vi "SCADA.vi"() -> ()   [LabVIEW 2014]
uses:
  <vilib>/Platform/TimedLoop/XDataNode/timing_clust.ctl
  <vilib>/Platform/TimedLoop/XDataNode/nitl_modes.ctl
  <vilib>/Platform/TimedLoop/XDataNode/wakeup.ctl
  <vilib>/platform/TimedLoop/XDataNode/XDataNode.xnode
  <vilib>/Platform/TimedLoop/XDataNode/XDNodeRunTimeDep.lvlib
panel:
  in  "SCADA":enum32{"Control panel", "Ulazi", "Izlazi"}(tab)
  in  "Stop SCADA":bool
  in  "On-Off":bool
  in  "Start":bool
  in  "Stop":bool
  in  "Fault":bool
  in  "Emergency Stop":bool
  in  "H3":bool
  in  "H4":bool
  in  "H5":bool
  in  "H6":bool
  in  "H7":bool
  in  "H8":bool
  in  "H9":bool
  in  "K1":bool
  in  "K2":bool
  in  "K3":bool
  in  "K4":bool
  in  "K5":bool
  in  "K6":bool
  in  "K7":bool
  in  "S1":bool
  in  "S2":bool
  in  "S3":bool
  in  "B1":bool
  in  "B2":bool
  in  "B3":bool
  in  "B4":bool
  in  "B5":bool
  in  "B6":bool
  in  "B7":bool
  in  "B8":bool
  in  "B9":bool
  in  "B10":bool
  in  "B11":bool
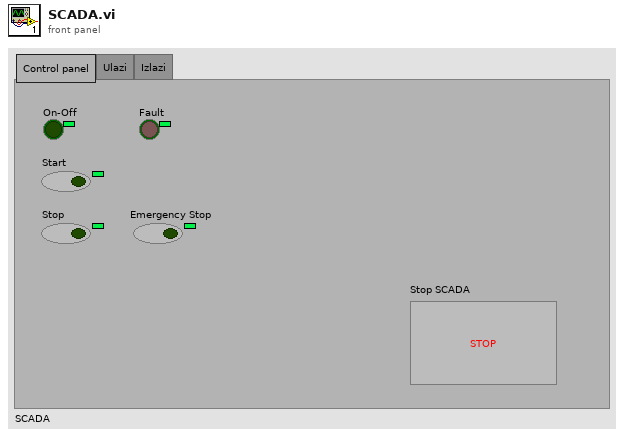
[diagram p1: front panel]
types:
  T1 = typedef "XDNodeRunTimeDep.lvlib/timing_clust.ctl" = cluster{"Expected End [f-1]":u64, "Actual End [f-1]":u64, "Finished Late? [f-1]":bool, "Expected End [i-1]":u64, "Actual End [i-1]":u64, "Finished Late? [i-1]":bool, "Expected Start [i]":u64, "Actual Start [i]":u64, "Expected Start [f]":u64, "Actual Start [f]":u64, "Source Name":string, "Structure Name":string, "Period":i64, "Deadline":i64, "Offset":i64, "Start":i64, "Priority":i32, "Timeout":i32, "Mode":T2, "Wakeup Reason":T3, "Error":errorcluster, "Source Type":string, "Secondary Source Type":string, "Global End Time":u64, "Global Start Time":u64, "Frame Duration":u64, "Iteration Duration":u64, "Assigned CPU":i32, "I/O Scan Engine Mode":u32}
  T2 = typedef "XDNodeRunTimeDep.lvlib/nitl_modes.ctl" = enum32{"No Change", "Process missed periods, maintain original phase", "Discard missed periods, maintain original phase", "Process missed periods, ignore original phase", "Discard missed periods, ignore original phase"}
  T3 = typedef "XDNodeRunTimeDep.lvlib/wakeup.ctl" = enum32{"Normal", "Aborted", "Asynchronous wakeup", "Timing source error", "Timed loop error", "Timeout"}
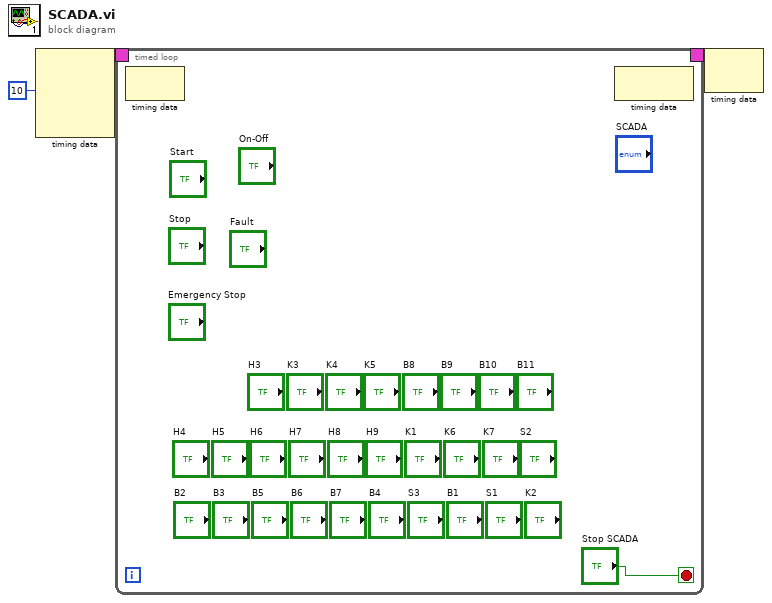
[diagram p0: block diagram]
diagram:
  n1 = node-c288(i64 10 ("Period")) -> (w3:T1)  [unwired: 3 in]
  n2 = timed-loop {
    timing: w3 -> [_]
    timing-out: [_] -> w2
    stop <- "Stop SCADA" stop-if-true
    n3 = node-c288() -> ()  [unwired: 1 in, 1 out]
    n4 = node-c288() -> ()  [unwired: 1 in, 1 out]
  }
  n5 = node-c288(w2) -> ()  [unwired: 1 out]
